vi "Test Broken.vi"(11 "Test Case In":refnum<class "Broken Test.lvclass">) -> (0 "error out":errorcluster, 3 "Test Case Out":refnum<class "Broken Test.lvclass">)   [LabVIEW 2020, in "Broken Test.lvclass"]
uses:
  Broken Test.lvclass
  e14b8b0a-9b7b-4cf5-9f85-09c4314edb9a.vi
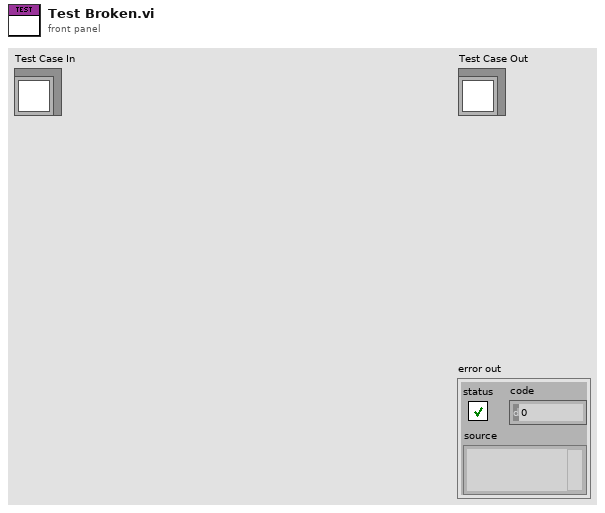
[diagram p1: front panel]
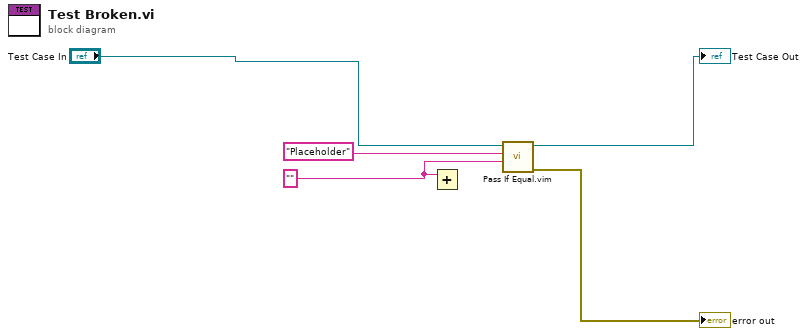
[diagram p0: block diagram]
diagram:
  w1 = ""
  n1 = Add(x=w1) -> ()  [unwired: 1 in, 1 out]
  n2 = call "Pass If Equal.vim"("Actual"=w1, "Expected"="Placeholder", "LUnit Test Case In"="Test Case In") -> ("error out"=→"error out":errorcluster, "LUnit Test Case Out"=→"Test Case Out":refnum<class "Broken Test.lvclass">)  [unwired: 7 in]
